vi "Write connection reference.vi"(8 "error in (no error)":errorcluster, 10 "reference":T1, 11 "DBMS in":refnum<class "DBMS.lvclass">) -> (0 "error out":errorcluster, 3 "DBMS out":refnum<class "DBMS.lvclass">)   [LabVIEW 2020, in "DBMS.lvclass"]
uses:
  DBMS.lvclass
  <vilib>/addons/database/Connection.llb/Conn ObjectReference.ctl
  DBMS.lvclass/DBMS.ctl
  <vilib>/addons/database/NI_Database_API.lvlib
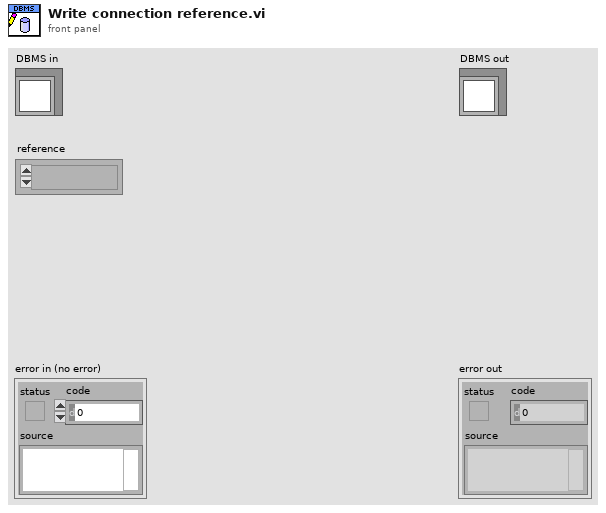
[diagram p1: front panel]
types:
  T1 = typedef "NI_Database_API.lvlib/Conn ObjectReference.ctl" = refnum<k1>
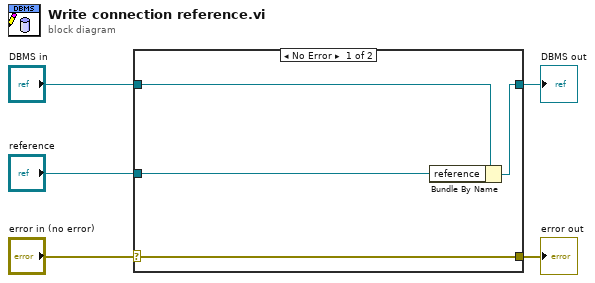
[diagram p0: block diagram]
diagram:
  n1 = case shown="No Error" "error in (no error)" {
    selector: "error in (no error)" -> [w9 w10]
    tunnel: [w9 w10] -> w4
    tunnel: [w7 w11] -> w2
    tunnel: "DBMS in" -> [w8 w11]
    tunnel: "reference" -> [w6 _]
    frame No Error {
      n2 = Bundle By Name(cluster=w8, "reference"=w6) -> (w7:refnum<class "DBMS.lvclass">)
    }
    frame Error {
    }
  }
  "error out" <- w4
  "DBMS out" <- w2
